vi "InstallerBuildSpec.SaveAndClose.vi"(8 "error in (no error)":errorcluster, 11 "InstallerMutationSession":T1={"Installer Build Specification Ref"=refnum, "Project reference out"=refnum, "Installer Project Path"=path "C:/Users/Public/Documents/Git-Source/VeriStand-Custom-Steps-For-TestStand/Source/LabVIEW Code/Installer/Installer - Copy.lvproj"}) -> (0 "error out":errorcluster={"status"=TRUE, "code"=7, "source"="Invoke Node in InstallerBuildSpec.OpenReference.vi\n<APPEND>\nMethod Name: <b>Project:Open</b>"})   [LabVIEW 2013, in "VeriStand Steps Version Mutation.lvlib"]
uses:
  VeriStand Steps Version Mutation.lvlib
  Types/LVInstallerMutationSession.ctl
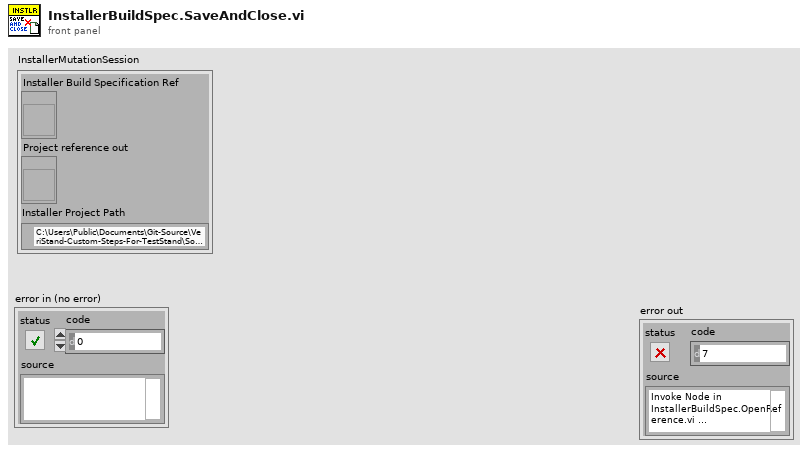
[diagram p1: front panel]
types:
  T1 = typedef "VeriStand Steps Version Mutation.lvlib/LVInstallerMutationSession.ctl" = cluster{"Installer Build Specification Ref":refnum<vi>, "Project reference out":refnum<vi>, "Installer Project Path":path}
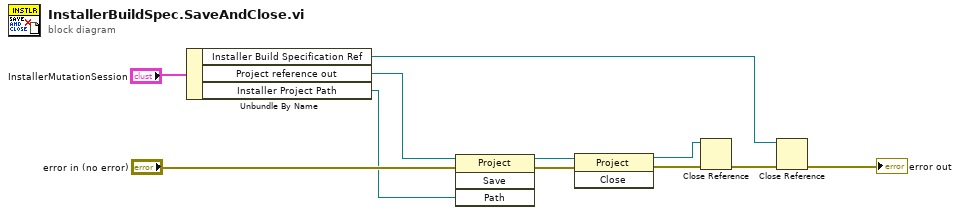
[diagram p0: block diagram]
diagram:
  n1 = Unbundle By Name("InstallerMutationSession") -> ("Installer Build Specification Ref"=w1:refnum<vi>, "Project reference out"=w3:refnum<vi>, "Installer Project Path"=w2:path)
  n2 = invoke class="Project" method="Save"(reference=w3, error in="error in (no error)", "Path"=w2) -> (reference out=w10:refnum<vi>, error out=w9:errorcluster)  [unwired: 1 in, 2 out]
  n3 = invoke class="Project" method="Close"(reference=w10, error in=w9) -> (reference out=w6:refnum<vi>, error out=w8:errorcluster)  [unwired: 1 in, 1 out]
  n4 = Close Reference(reference=w6, error in (no error)=w8) -> (error out=w7:errorcluster)
  n5 = Close Reference(reference=w1, error in (no error)=w7) -> (error out=→"error out":errorcluster)
